vi "Random Main Question.vi"(4 "Answer":T2, 6 "Fist Run?":bool) -> (1 "Question Index":T1, 2 "End":bool, 3 "AI Question":string)   [LabVIEW 2015]
uses:
  Data Def/Answer.ctl
  Data Def/Question Index.ctl
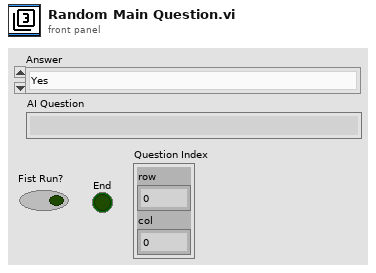
[diagram p1: front panel]
types:
  T1 = typedef "Question Index.ctl" = cluster{"row":i32, "col":i32}
  T2 = typedef "Answer.ctl" = enum16{"Yes", "No", "I don't Know"}
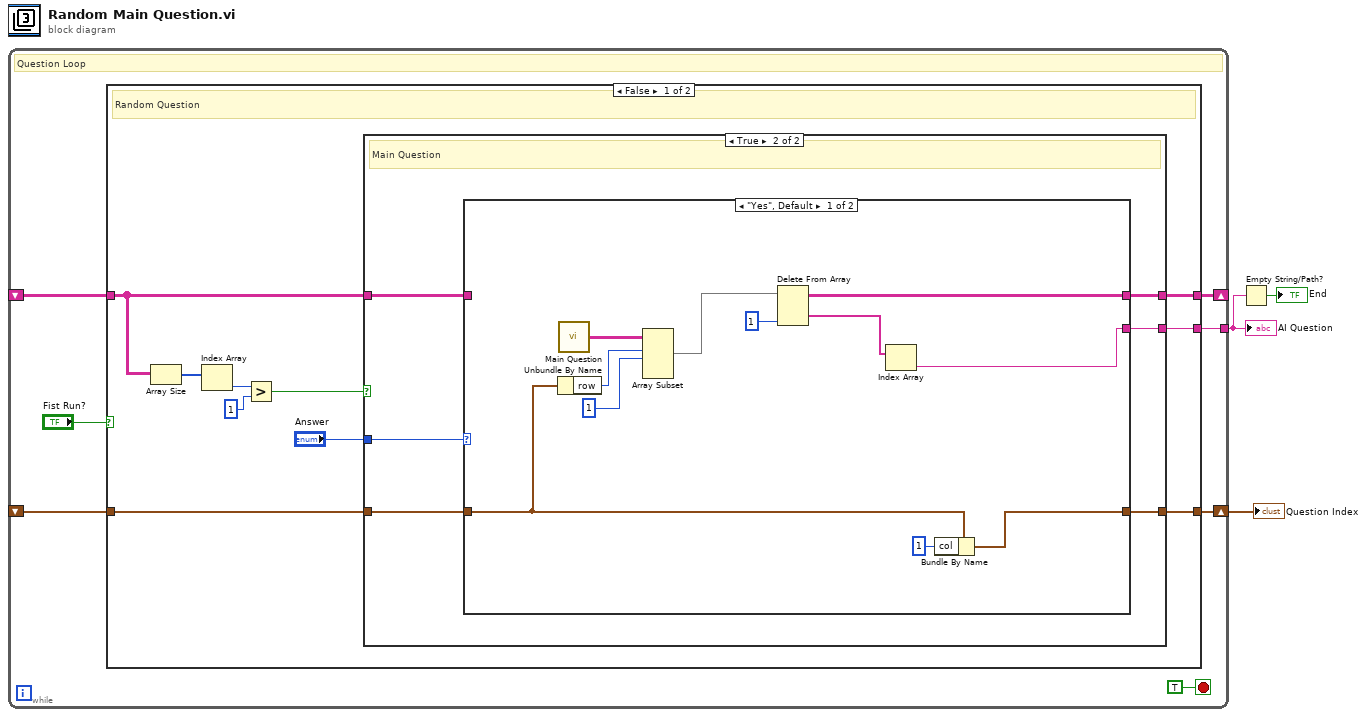
[diagram p0: block diagram]
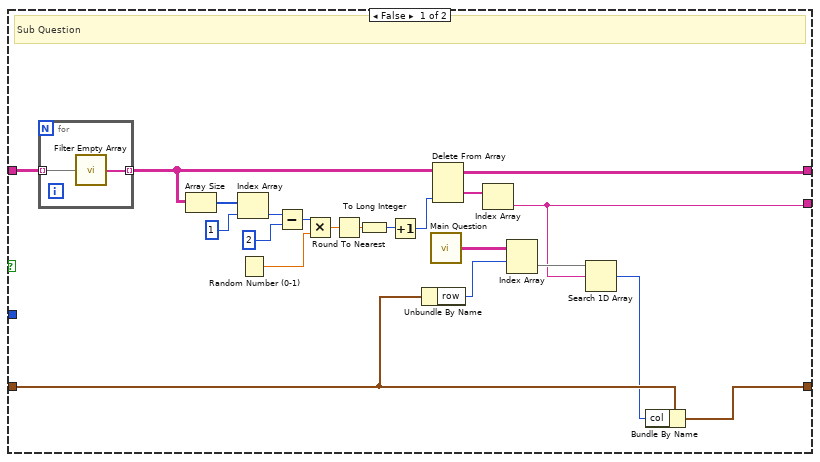
[diagram p2: hidden frame]
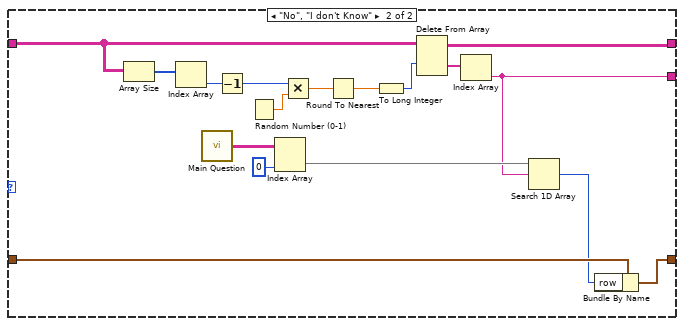
[diagram p3: hidden frame]
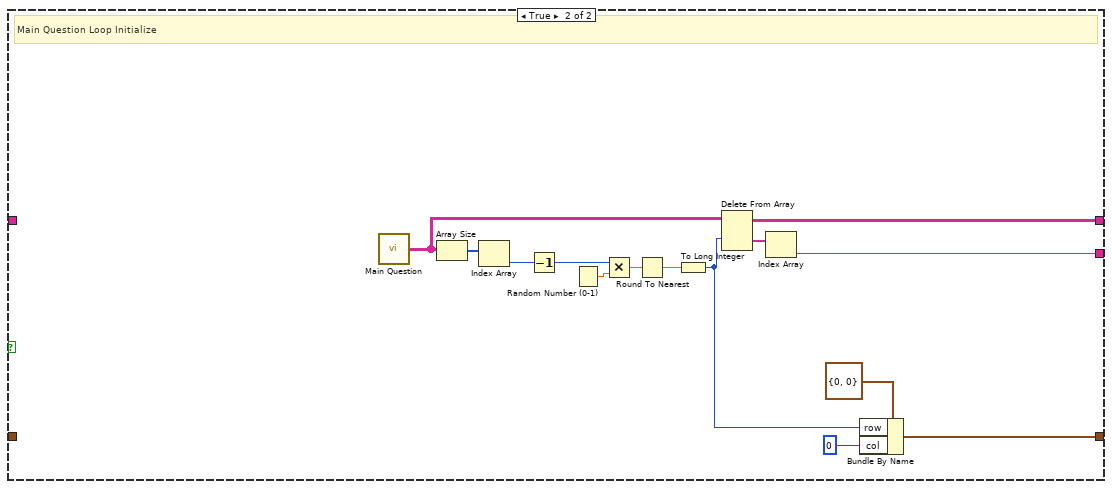
[diagram p4: hidden frame]
diagram:
  n1 = while {
    shift-right: [w8] -> _
    shift-left: _ -> [w6]
    tunnel: [w7] -> w1
    shift-right: [w5] -> w2
    shift-left: _ -> [w4]
    stop <- TRUE stop-if-true
    # "Question Loop"
    n2 = case shown="False" "Fist Run?" {
      tunnel: [w20 w85] -> w8
      tunnel: [w19 w83] -> w7
      tunnel: w6 -> [w18 _]
      tunnel: [w12 w81] -> w5
      tunnel: w4 -> [w11 _]
      frame False {
        # "Random Question"
        n3 = Array Size(array=w18) -> (size(s)=w17:i32[])
        n4 = Index Array(array=w17) -> (element=w16:i32)  [unwired: 1 in]
        n5 = Greater?(x=w16, y=1) -> (0:w14:bool)
        n6 = case shown="True" w14 {
          tunnel: w18 -> [w28 w49]
          tunnel: [w21 w48] -> w20
          tunnel: [w30 w47] -> w19
          tunnel: "Answer" -> [_ w46]
          tunnel: [w40 w45] -> w12
          tunnel: w11 -> [w34 w44]
          frame False {
            # "Sub Question"
            n7 = for {
              tunnel: w28 -> [w43] mode=indexing
              tunnel: [w42] -> w27 mode=indexing
              n8 = call "Filter Empty Array.vi"("Array In"=w43) -> ("Array Out"=w42:string[])
            }
            n9 = Array Size(array=w27) -> (size(s)=w36:i32[])
            n10 = Index Array(array=w36, index=1) -> (element=w26:i32)
            n11 = Random Number (0-1)() -> (number: 0 to 1=w39:dbl)
            n12 = Subtract(x=w26, y=2) -> (x-y=w25:i32)
            n13 = Multiply(x=w25, y=w39) -> (x*y=w38:dbl)
            n14 = Round To Nearest(number=w38) -> (nearest integer value=w37:dbl)
            n15 = To Long Integer(number=w37) -> (32bit integer=w23:i32)
            n16 = Increment(x=w23) -> (x+1=w22:i32)
            n17 = Unbundle By Name(w34) -> ("row"=w32:i32)
            n18 = call "Main Question.vi"() -> ("Question"=w33:string[][])
            n19 = Delete From Array(array=w27, index (col)=w22) -> (deleted portion=w41:string[], array with subset deleted=w21:string[][])  [unwired: 2 in]
            n20 = Index Array(array=w41) -> (element=w30:string)  [unwired: 1 in]
            n21 = Index Array(array=w33, index (row)=w32) -> (element=w31:string[])  [unwired: 1 in]
            n22 = Search 1D Array(1D array=w31, element=w30) -> (index of element=w29:i32)  [unwired: 1 in]
            n23 = Bundle By Name(cluster=w34, "col"=w29) -> (w40:T1)
          }
          frame True {
            # "Main Question"
            n24 = case shown="\"Yes\", Default" w46 {
              tunnel: w49 -> [_ w70]
              tunnel: [w50 w69] -> w48
              tunnel: [w54 w62] -> w47
              tunnel: [w59 w68] -> w45
              tunnel: w44 -> [w58 w66]
              frame "Yes", Default {
                n25 = Unbundle By Name(w58) -> ("row"=w56:i32)
                n26 = call "Main Question.vi"() -> ("Question"=w57:string[][])
                n27 = Array Subset(array=w57, index (row)=w56, length (row)=1 ("length")) -> (w53:string[][])  [unwired: 2 in]
                n28 = Delete From Array(array=w53, index (col)=1 ("disabled index (col)")) -> (deleted portion=w51:string[], array with subset deleted=w50:string[][])  [unwired: 2 in]
                n29 = Index Array(array=w51) -> (element=w54:string)  [unwired: 1 in]
                n30 = Bundle By Name(cluster=w58, "col"=1) -> (w59:T1)
              }
              frame "No", "I don't Know" {
                n31 = Array Size(array=w70) -> (size(s)=w73:i32[])
                n32 = Index Array(array=w73) -> (element=w72:i32)  [unwired: 1 in]
                n33 = call "Main Question.vi"() -> ("Question"=w65:string[][])
                n34 = Decrement(x=w72) -> (x-1=w77:i32)
                n35 = Random Number (0-1)() -> (number: 0 to 1=w76:dbl)
                n36 = Index Array(array=w65, index (col)=0 ("disabled index (col)")) -> (element=w63:string[])  [unwired: 1 in]
                n37 = Multiply(x=w77, y=w76) -> (x*y=w75:dbl)
                n38 = Round To Nearest(number=w75) -> (nearest integer value=w74:dbl)
                n39 = To Long Integer(number=w74) -> (32bit integer=w67:i32)
                n40 = Delete From Array(array=w70, index (row)=w67) -> (deleted portion=w71:string[], array with subset deleted=w69:string[][])  [unwired: 2 in]
                n41 = Index Array(array=w71) -> (element=w62:string)  [unwired: 1 in]
                n42 = Search 1D Array(1D array=w63, element=w62) -> (index of element=w61:i32)  [unwired: 1 in]
                n43 = Bundle By Name(cluster=w66, "row"=w61) -> (w68:T1)
              }
            }
          }
        }
      }
      frame True {
        # "Main Question Loop Initialize"
        n44 = call "Main Question.vi"() -> ("Question"=w78:string[][])
        n45 = Array Size(array=w78) -> (size(s)=w87:i32[])
        n46 = Index Array(array=w87) -> (element=w86:i32)  [unwired: 1 in]
        n47 = Decrement(x=w86) -> (x-1=w91:i32)
        n48 = Random Number (0-1)() -> (number: 0 to 1=w90:dbl)
        n49 = Multiply(x=w91, y=w90) -> (x*y=w89:dbl)
        n50 = Round To Nearest(number=w89) -> (nearest integer value=w88:dbl)
        n51 = To Long Integer(number=w88) -> (32bit integer=w80:i32)
        n52 = Delete From Array(array=w78, index (row)=w80) -> (deleted portion=w84:string[], array with subset deleted=w85:string[][])  [unwired: 2 in]
        n53 = Index Array(array=w84) -> (element=w83:string)  [unwired: 1 in]
        n54 = Bundle By Name(cluster=T1 {"row"=0, "col"=0}, "row"=w80, "col"=0) -> (w81:T1)
      }
    }
  }
  "AI Question" <- w1
  "Question Index" <- w2
  n55 = Empty String/Path?(string/path=w1) -> (empty?=→"End":bool)
